vi "ReadStream ServerStreamTemplate.vi"(8 "error in":errorcluster, 11 "Call ID in":T1) -> (0 "error out":errorcluster, 1 "Success":bool, 2 "Response Data":cluster{"Numeric":dbl}, 3 "Call ID":T1)   [LabVIEW 2019, in "Client Template.lvlib"]
uses:
  Client Template.lvlib
  <vilib>/gRPC/LabVIEW gRPC Library/Shared/grpcId.ctl
  aea5dbbb-03a2-479b-ad95-94da4ee1cea9.vi
  <vilib>/gRPC/LabVIEW gRPC Library/Shared/TranslateGrpcError.vi
  <vilib>/gRPC/LabVIEW gRPC Library/Shared/Wait On Occurence.vi
  <vilib>/AdvancedString/1D String Array to Delimited String.vi
  <vilib>/gRPC/LabVIEW gRPC Library/Server API/Server/Get Server DLL Path.vi
  <vilib>/gRPC/LabVIEW gRPC Library/grpc-lvsupport-release.lvlib
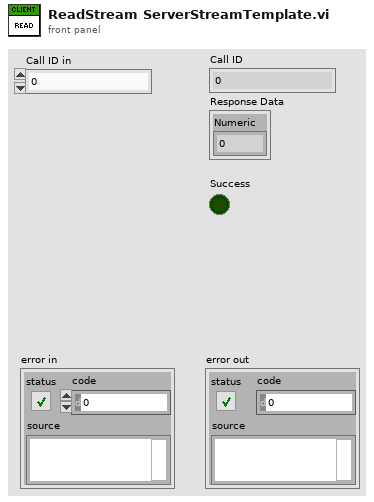
[diagram p1: front panel]
types:
  T1 = typedef "grpc-lvsupport-release.lvlib/grpcId.ctl" = u64
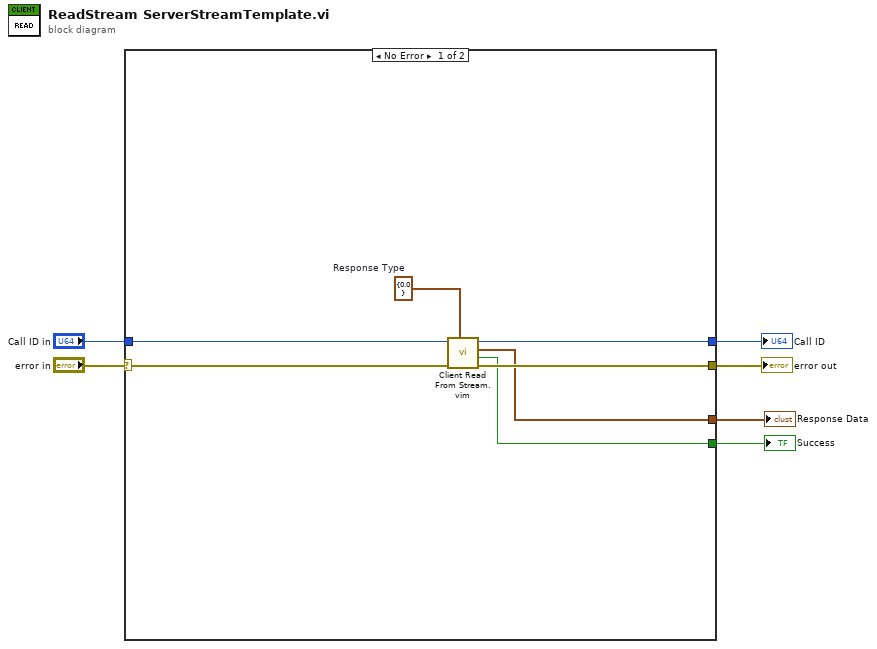
[diagram p0: block diagram]
diagram:
  n1 = case shown="No Error" "error in" {
    selector: "error in" -> [w13 w14]
    tunnel: [w12 w14] -> w5
    tunnel: "Call ID in" -> [w11 w15]
    tunnel: [w7 w15] -> w3
    tunnel: [w10 _] -> w2
    tunnel: [w8 _] -> w1
    frame No Error {
      w9 = cluster{"Numeric":dbl} {"Numeric"=0.0}  # Response Type
      n2 = call "Client Read From Stream.vim"("Response Type"=w9, "error in"=w13, "Call ID in"=w11) -> ("error out"=w12:errorcluster, "Success"=w8:bool, "Response Data"=w10:cluster{"Numeric":dbl}, "Call ID out"=w7:u64)  [unwired: 5 in]
    }
    frame Error {
    }
  }
  "error out" <- w5
  "Call ID" <- w3
  "Response Data" <- w2
  "Success" <- w1
